vi "Serialize.vi"(8 "error in (no error)":errorcluster, 11 "VIConverter in":refnum<class "VIConverter.lvclass">) -> (0 "error out":errorcluster, 2 "JSON":string, 3 "VIConverter out":refnum<class "VIConverter.lvclass">)   [LabVIEW 2017]
uses:
  JSONConstants.vi
  SupportedFileTypes.ctl
  VIConverter.lvclass
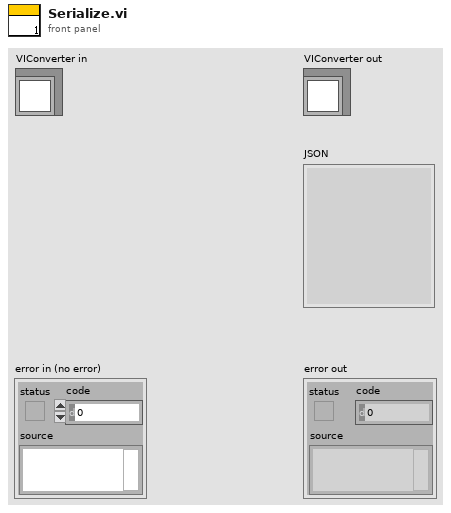
[diagram p1: front panel]
types:
  T1 = typedef "SupportedFileTypes.ctl" = enum16{"VirtualInstrument", "Class", "Project"}
  T2 = enum32{"invalid VI type", "Standard VI", "Control VI", "Global VI", "Polymorphic VI", "Configuration VI", "SubSystem", "Facade VI", "Method VI", "Statechart Diagram VI"}
  T3 = cluster{"VIPath":path, "Menu Name":string, "Selector Name":string}[]
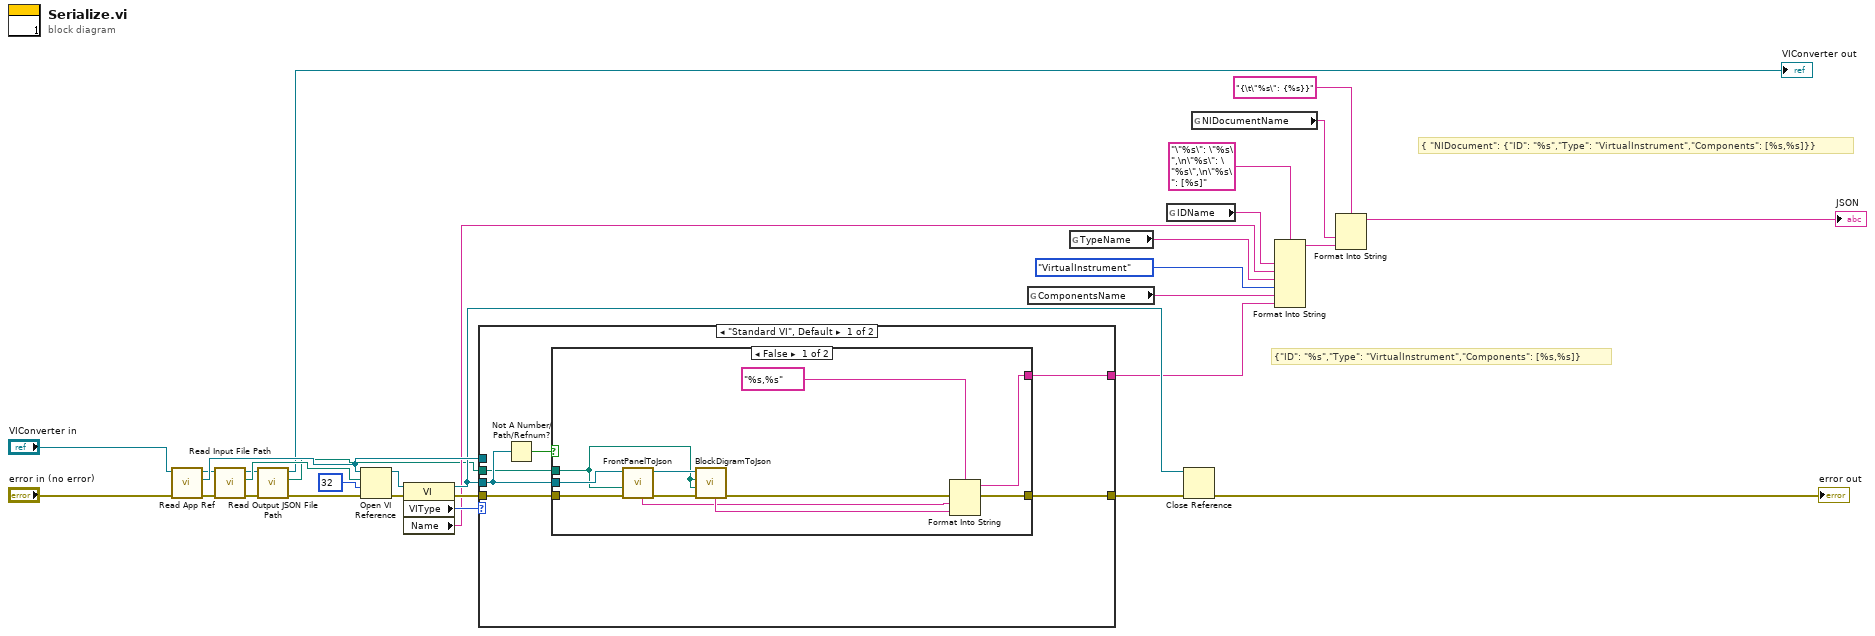
[diagram p0: block diagram]
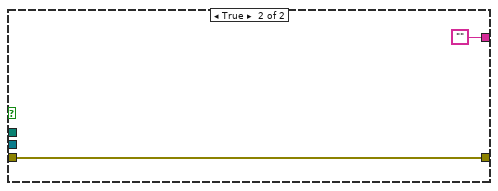
[diagram p2: hidden frame]
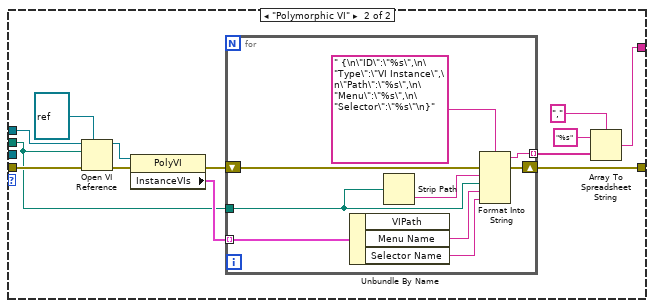
[diagram p3: hidden frame]
diagram:
  # "{\t\"NIDocument\": {\"ID\": \"%s\",\"Type\": \"VirtualInstrument\",\"Components\": [%s,%s]}}"
  # "{\"ID\": \"%s\",\"Type\": \"VirtualInstrument\",\"Components\": [%s,%s]}"
  n1 = call-dynamic "Read App Ref.vi"("error in (no error)"="error in (no error)", "FileConverterBase in"="VIConverter in") -> ("error out"=w22:errorcluster, "App Ref"=w24:refnum<vi>, "FileConverterBase out"=w21:refnum<class "VIConverter.lvclass">)  [unwired: 7 in]
  n2 = call-dynamic "Read Input File Path.vi"("error in (no error)"=w22, "FileConverterBase in"=w21) -> ("error out"=w5:errorcluster, "Input File Path"=w20:path, "FileConverterBase out"=w3:refnum<class "VIConverter.lvclass">)  [unwired: 7 in]
  n3 = call-dynamic "Read Output JSON File Path.vi"("error in (no error)"=w5, "FileConverterBase in"=w3) -> ("error out"=w1:errorcluster, "Output JSON File Path"=w4:path, "FileConverterBase out"=→"VIConverter out":refnum<class "VIConverter.lvclass">)  [unwired: 7 in]
  n4 = Open VI Reference(application reference (local)=w24, vi path=w20, options=32, error in (no error)=w1) -> (vi reference=w30:refnum<vi>, error out=w29:errorcluster)  [unwired: 2 in]
  n5 = property class="VI"(reference=w30, error in=w29) -> (reference out=w17:refnum<vi>, error out=w28:errorcluster, "VIType"=w26:T2, "Name"=w10:string)
  n6 = case shown="\"Standard VI\", Default" w26 {
    tunnel: [w36 w55] -> w19
    tunnel: w28 -> [w33 w53]
    tunnel: w17 -> [w34 _]
    tunnel: w24 -> [_ w52]
    tunnel: [w32 w51] -> w6
    tunnel: w4 -> [w31 w50]
    frame "Standard VI", Default {
      n7 = Not A Number/Path/Refnum?(number/path/refnum=w34) -> (NaN/Path/Refnum?=w35:bool)
      n8 = case shown="False" w35 {
        tunnel: [w40 w49] -> w36
        tunnel: w33 -> [w38 w49]
        tunnel: w34 -> [w47 _]
        tunnel: [w39 ""] -> w32
        tunnel: w31 -> [w37 _]
        frame False {
          n9 = call "FrontPanelToJson.vi"("error in"=w38, "JSON Path"=w37, "VI in"=w47) -> ("error out"=w45:errorcluster, "VI out"=w43:refnum<vi>, "JSON"=w41:string)  [unwired: 5 in]
          n10 = call "BlockDigramToJson.vi"("error in"=w45, "origin path"=w37, "created path"=w37, "VI in"=w43) -> ("error out"=w44:errorcluster, "JSON"=w42:string)  [unwired: 4 in, 1 out]
          n11 = Format Into String(format string="%s,%s", error in=w44, w41, w42) -> (resulting string=w39:string, error out=w40:errorcluster)  [unwired: 1 in]
        }
        frame True {
        }
      }
    }
    frame "Polymorphic VI" {
      n12 = Open VI Reference(type specifier VI Refnum (for type only)=refnum<vi> refnum, application reference (local)=w52, vi path=w50, error in (no error)=w53) -> (vi reference=w61:refnum<vi>, error out=w56:errorcluster)  [unwired: 2 in]
      n13 = property class="PolyVI"(reference=w61, error in=w56) -> (error out=w54:errorcluster, "InstanceVIs"=w60:T3)  [unwired: 1 out]
      n14 = for {
        tunnel: w60 -> [w71] mode=indexing
        tunnel: [w67] -> w59 mode=indexing
        shift-right: [w65] -> w55
        shift-left: w54 -> [w64]
        tunnel: w50 -> [w63]
        n15 = Unbundle By Name(w71) -> ("Menu Name"=w69:string, "Selector Name"=w68:string)  [unwired: 1 out]
        n16 = Strip Path(path=w63) -> (name=w66:string)  [unwired: 1 out]
        n17 = Format Into String(format string=" {\n\"ID\":\"%s\",\n\"Type\":\"VI Instance\",\n\"Path\":\"%s\",\n\"Menu\":\"%s\",\n\"Selector\":\"%s\"\n}", error in=w64, w66, w63, w69, w68) -> (resulting string=w67:string, error out=w65:errorcluster)  [unwired: 1 in]
      }
      n18 = Array To Spreadsheet String(delimiter (Tab)=",", array=w59, 3:"%s" ("format string")) -> (spreadsheet string=w51:string)
    }
  }
  n19 = global read "JSONConstants.vi" "ComponentsName"() -> (w7:string)
  n20 = global read "JSONConstants.vi" "TypeName"() -> (w9:string)
  n21 = global read "JSONConstants.vi" "IDName"() -> (w11:string)
  n22 = Close Reference(reference=w17, error in (no error)=w19) -> (error out=→"error out":errorcluster)
  n23 = global read "JSONConstants.vi" "NIDocumentName"() -> (w15:string)
  n24 = Format Into String(format string="\"%s\": \"%s\",\n\"%s\": \"%s\",\n\"%s\": [%s]", w11, w10, w9, SupportedFileTypes."VirtualInstrument" ("Supported File Types"), w7, w6) -> (resulting string=w13:string)  [unwired: 2 in, 1 out]
  n25 = Format Into String(format string="{\t\"%s\": {%s}}", w15, w13) -> (resulting string=→"JSON":string)  [unwired: 2 in, 1 out]
